vi "Set_PS1_15V_independent.vi"(3 "error in":errorcluster) -> (10 "error out":errorcluster)   [LabVIEW 2015]
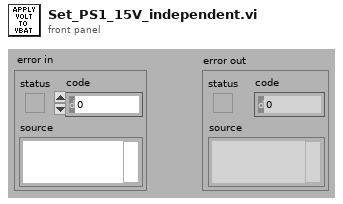
[diagram p1: front panel]
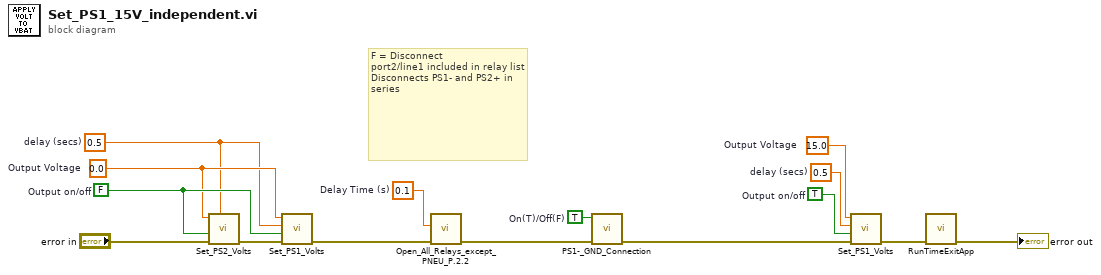
[diagram p0: block diagram]
diagram:
  w1 = 0.1  # Delay Time (s)
  w2 = TRUE  # On(T)/Off(F)
  w11 = TRUE  # Output on/off
  w10 = 0.5  # delay (secs)
  w9 = 15.0  # Output Voltage
  w13 = 0.0  # Output Voltage
  w12 = 0.5  # delay (secs)
  w14 = FALSE  # Output on/off
  # "F = Disconnect\nport2/line1 included in relay list \nDisconnects PS1- and PS2+ in series"
  n1 = call "Set_PS2_Volts.vi"("delay (secs)"=w12, "error in"="error in", "Output on/off"=w14, "Output Voltage"=w13) -> ("error out"=w15:errorcluster)  [unwired: 5 in, 2 out]
  n2 = call "Set_PS1_Volts.vi"("error in"=w15, "Output on/off"=w14, "delay (secs)"=w12, "Output Voltage"=w13) -> ("error out"=w7:errorcluster)  [unwired: 5 in, 2 out]
  n3 = call "Open_All_Relays_except_PNEU_P.2.2.vi"("Delay Time (s)"=w1, "error in"=w7) -> ("error out"=w4:errorcluster)  [unwired: 8 in]
  n4 = call "PS1-_GND_Connection.vi"("On/Off"=w2, "error in"=w4) -> ("error out"=w3:errorcluster)  [unwired: 8 in]
  n5 = call "Set_PS1_Volts.vi"("error in"=w3, "Output on/off"=w11, "delay (secs)"=w10, "Output Voltage"=w9) -> ("error out"=w8:errorcluster)  [unwired: 5 in, 2 out]
  n6 = call "RunTimeExitApp.vi"("error in (no error)"=w8) -> ("error out"=→"error out":errorcluster)  [unwired: 10 in]
